vi "PatientSpecificFileNameGen.vi"(3 "Auto Increment":bool, 4 "Done":bool, 5 "Add to Database":bool) -> (0 "SavePathOut":path, 1 "PatientFileName":string)   [LabVIEW 2022 SP3]
uses:
  Patient Routines/PatientGlobals.vi
  ScanningControl/Motion Controllers/-MotionRoutines/MotionGlobals.vi
  ViewData/-ReadEye/TypeDefs/TissueType.ctl
  Patient Routines/LymphNodeInfo.ctl
  Patient Routines/TissueTypeScan.ctl
panel:
  in  "Node Info":T1 {"Year" format="%02d"; "Patient Number" format="%03d"; "Node Number" format="%02d"}
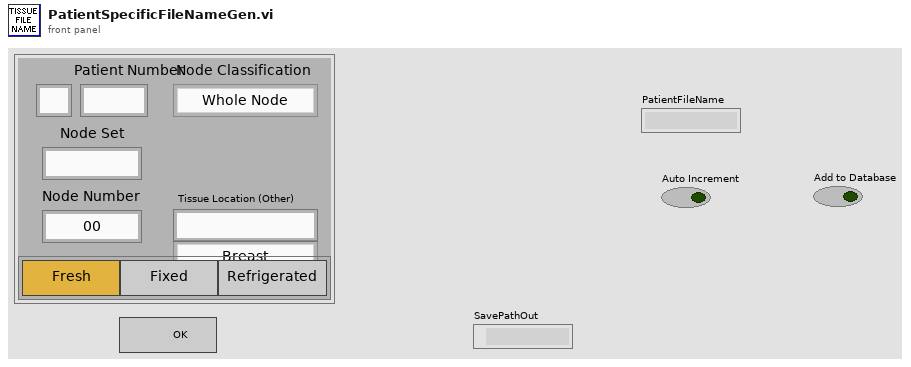
[diagram p1: front panel]
types:
  T1 = typedef "LymphNodeInfo.ctl" = cluster{"Patient Number":u32, "Node Set":string, "Node Number":u32, "Tissue Type":T2, "Tissue Location (Other)":string, "Node Classification":enum16{"Whole Node", "Piece A", "Piece B", "Piece C"}, "Fresh?":enum32{"Fresh?", "Fixed?", "Refrigerated?"}, "Year":u32}
  T2 = typedef "TissueTypeScan.ctl" = enum16{"Breast", "Gastric", "Stomach", "Rectal", "Colon", "Head & Neck", "Other"}
  T3 = typedef "location.ctl" = enum16{"Automatic", "WCM Main", "Hawaii", "Columbia MM3000", "Columbia  NI System", "NYU", "RRI 2", "UHI Allen", "CUMC RT", "Chiba", "Stony Brook", "WCM Microscopy", "WCM Aeoretch", "WCM Optics Lab", "WCM Main 2Axis", "WCM Rotation", "WCM SAM SMAC", "SERI GP"}
  T4 = enum16{"Whole Node", "Sentinel A", "Sentinel B", "Sentinel C"}
  T5 = typedef "TissueType.ctl" = enum16{"Breast", "Gastric", "Stomach", "Rectal", "Colon", "Head & Neck", "Other"}
  T6 = enum16{"open", "replace", "create", "open or create", "replace or create", "replace or create with confirmation"}
  T7 = typedef "TissueType.ctl" = cluster{"organ":i16, "disease type":i16, "disease location":i16, "IQ_pts":u16, "RcvBuffer":u8, "RcvFrame":u16, "IQBuff":u8, "IQFrame":u16, "IQPage":u8}
  T8 = enum16{"Whole Node", "Piece A", "Piece B", "Piece C"}
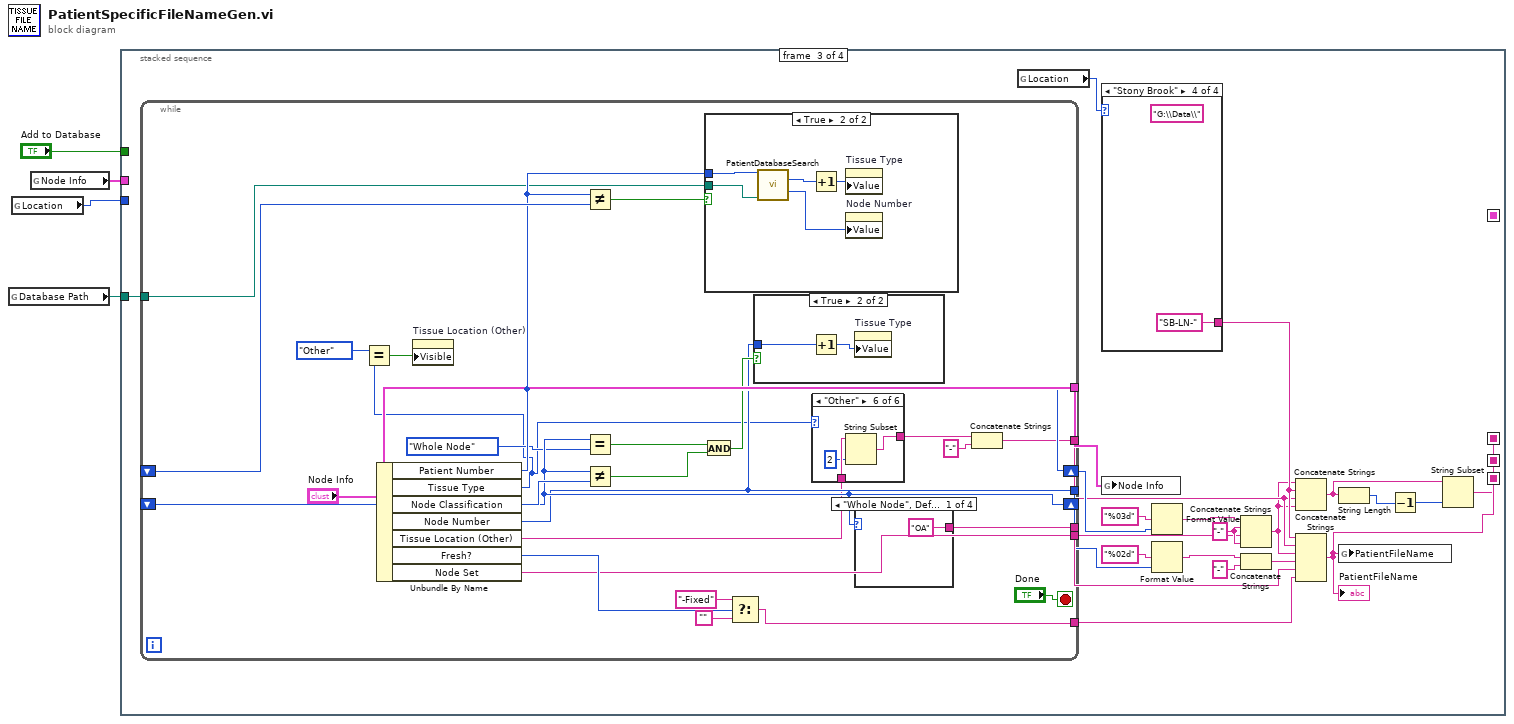
[diagram p0: block diagram]
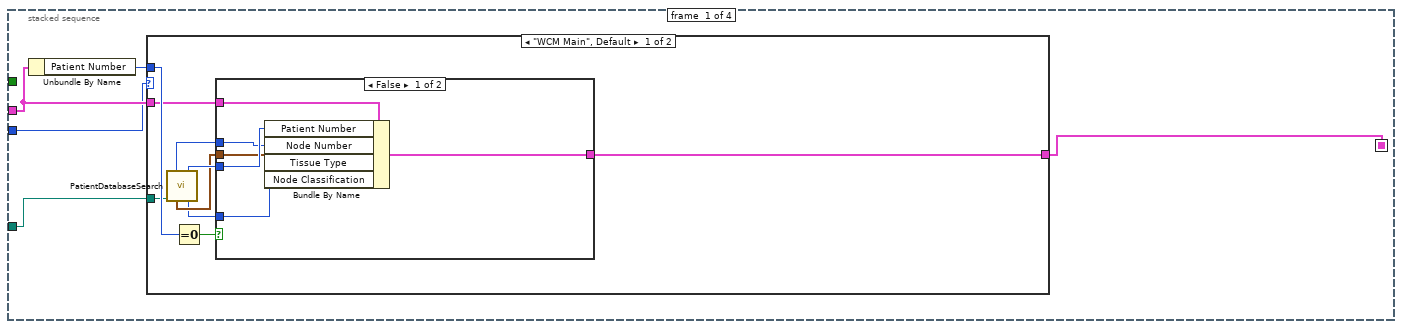
[diagram p2: hidden frame]
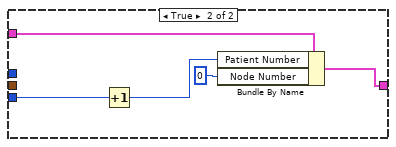
[diagram p3: hidden frame]
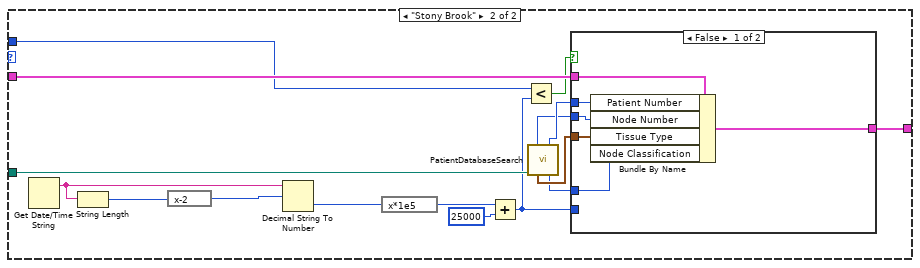
[diagram p4: hidden frame]
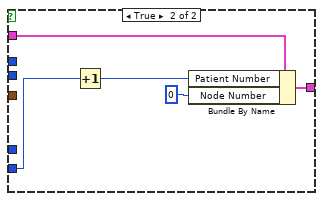
[diagram p5: hidden frame]
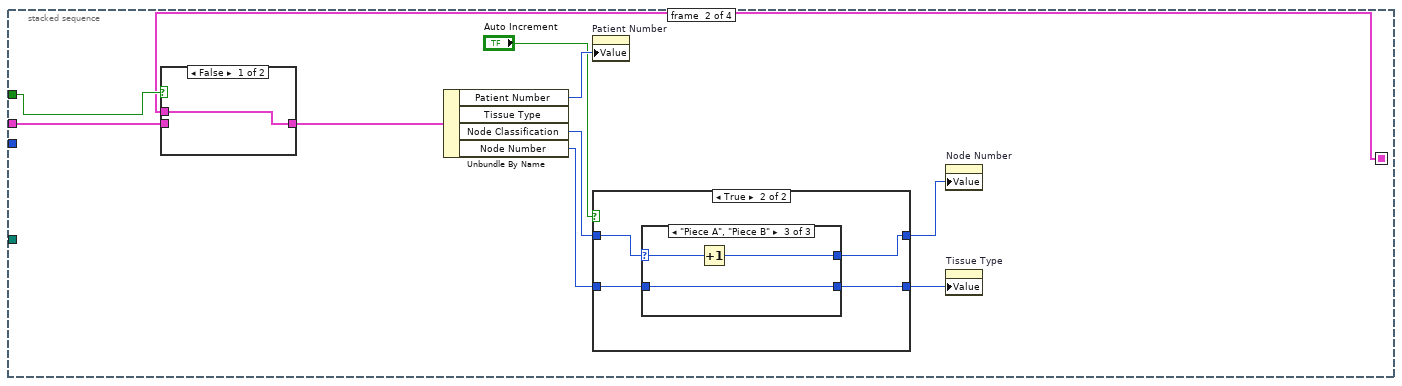
[diagram p6: hidden frame]
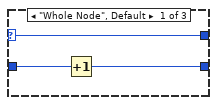
[diagram p9: hidden frame]
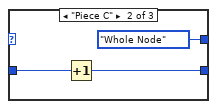
[diagram p10: hidden frame]
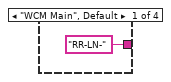
[diagram p11: hidden frame]
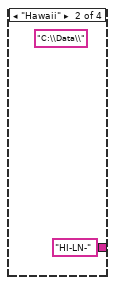
[diagram p12: hidden frame]
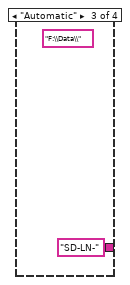
[diagram p13: hidden frame]
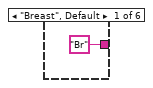
[diagram p16: hidden frame]
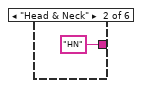
[diagram p17: hidden frame]
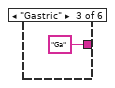
[diagram p18: hidden frame]
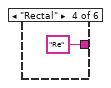
[diagram p19: hidden frame]
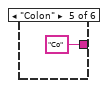
[diagram p20: hidden frame]
diagram:
  n1 = global read "PatientGlobals.vi" "Database Path"() -> (w4:path)
  n2 = global read "MotionGlobals.vi" "Location"() -> (w1:T3)
  n3 = global read "PatientGlobals.vi" "Node Info"() -> (w2:T1)
  n4 = stacked-sequence {
    seq-local: [_ _ w90 _] -> [_ _ _ w168]
    seq-local: [_ _ w101 _] -> [_ _ _ w166]
    seq-local: [_ _ w101 _] -> [_ _ _ w164]
    seq-local: [w6 _ _ _] -> [_ w57 _ _]
    tunnel: w4 -> [w8 _ w99 w163]
    tunnel: "Add to Database" -> [_ w60 _ w156]
    tunnel: w2 -> [w7 w59 _ _]
    tunnel: w1 -> [w5 _ _ _]
    frame #0 {
      n5 = Unbundle By Name(w7) -> ("Patient Number"=w9:u32)
      n6 = case shown="\"WCM Main\", Default" w5 {
        tunnel: w9 -> [w18 w38]
        tunnel: w8 -> [w16 w45]
        tunnel: w7 -> [w11 w40]
        tunnel: [w10 w39] -> w6
        frame "WCM Main", Default {
          n7 = call "PatientDatabaseSearch.vi"("file path (use dialog)"=w16) -> ("Last node of Last patient"=w14:i32, "Last Patient Number"=w15:i32, "Tissue Type of Last Node"=w13:T7, "Node Classification Of Last Patient"=w12:T4)  [unwired: 5 in, 6 out]
          n8 = Equal To 0?(x=w18) -> (x = 0?=w17:bool)
          n9 = case shown="False" w17 {
            tunnel: w11 -> [w24 w29]
            tunnel: w15 -> [w22 w27]
            tunnel: [w23 w25] -> w10
            tunnel: w14 -> [w21 _]
            tunnel: w13 -> [w20 _]
            tunnel: w12 -> [w19 _]
            frame False {
              n10 = Bundle By Name(cluster=w24, "Patient Number"=w22, "Node Number"=w21, "Tissue Type"=w20, "Node Classification"=w19) -> (w23:T1)
            }
            frame True {
              n11 = Increment(x=w27) -> (x+1=w28:i32)
              n12 = Bundle By Name(cluster=w29, "Patient Number"=w28, "Node Number"=u32 0) -> (w25:T1)
            }
          }
        }
        frame "Stony Brook" {
          n13 = Get Date/Time String() -> (date string=w35:string)  [unwired: 3 in, 1 out]
          n14 = String Length(string=w35) -> (length=w36:i32)
          n15 = expression code="x-2"(w36) -> (w34:i32)
          n16 = Decimal String To Number(string=w35, offset=w34) -> (number=w31:i32)  [unwired: 1 in, 1 out]
          n17 = expression code="x*1e5"(w31) -> (w30:i32)
          n18 = Add(x=w30, y=u32 25000) -> (x+y=w32:u32)
          n19 = Less?(x=w38, y=w32) -> (x < y?=w37:bool)
          n20 = call "PatientDatabaseSearch.vi"("file path (use dialog)"=w45) -> ("Last node of Last patient"=w43:i32, "Last Patient Number"=w44:i32, "Tissue Type of Last Node"=w42:T7, "Node Classification Of Last Patient"=w41:T4)  [unwired: 5 in, 6 out]
          n21 = case shown="False" w37 {
            tunnel: w40 -> [w51 w56]
            tunnel: w44 -> [w49 _]
            tunnel: [w50 w53] -> w39
            tunnel: w43 -> [w48 _]
            tunnel: w42 -> [w47 _]
            tunnel: w41 -> [w46 _]
            tunnel: w32 -> [_ w52]
            frame False {
              n22 = Bundle By Name(cluster=w51, "Patient Number"=w49, "Node Number"=w48, "Tissue Type"=w47, "Node Classification"=w46) -> (w50:T1)
            }
            frame True {
              n23 = Increment(x=w52) -> (x+1=w55:u32)
              n24 = Bundle By Name(cluster=w56, "Patient Number"=w55, "Node Number"=u32 0) -> (w53:T1)
            }
          }
        }
      }
    }
    frame #1 {
      n25 = case shown="False" w60 {
        tunnel: [w67 w68] -> w58
        tunnel: w59 -> [_ w68]
        tunnel: w57 -> [w67 _]
        frame False {
        }
        frame True {
        }
      }
      n26 = Unbundle By Name(w58) -> ("Patient Number"=w65:u32, "Node Classification"=w63:T8, "Node Number"=w64:u32)  [unwired: 1 out]
      n27 = property on="Patient Number" class="DigNum (strict)"("Value"=w65) -> ()  [unwired: 2 in, 2 out]
      n28 = case shown="True" "Auto Increment" {
        tunnel: [w69 w74] -> w66
        tunnel: w64 -> [w69 w73]
        tunnel: w63 -> [w70 w72]
        tunnel: [w70 w71] -> w62
        frame False {
        }
        frame True {
          n29 = case shown="\"Piece A\", \"Piece B\"" w72 {
            selector: w72 -> [w75 _ w82]
            tunnel: [w77 w78 w83] -> w74
            tunnel: w73 -> [w76 w79 w83]
            tunnel: [w75 T4."Whole Node" ("Node Classification") w81] -> w71
            frame "Whole Node", Default {
              n30 = Increment(x=w76) -> (x+1=w77:u32)
            }
            frame "Piece C" {
              n31 = Increment(x=w79) -> (x+1=w78:u32)
            }
            frame "Piece A", "Piece B" {
              n32 = Increment(x=w82) -> (x+1=w81:T8)
            }
          }
        }
      }
      n33 = property on="Node Number" class="DigNum (strict)"("Value"=w62) -> ()  [unwired: 2 in, 2 out]
      n34 = property on="Tissue Type" class="Enum (strict)"("Value"=w66) -> ()  [unwired: 2 in, 2 out]
    }
    frame #2 {
      w85 = "-" ("string")
      n35 = while {
        tunnel: [w121] -> w96
        tunnel: [w134] -> w102
        shift-right: [w130] -> w104
        shift-left: _ -> [w132]
        tunnel: ["Node Info"] -> w103
        tunnel: w99 -> [w129]
        shift-right: [w126] -> _
        shift-left: _ -> [w128]
        tunnel: [w122] -> w98
        tunnel: [w119] -> w86
        tunnel: [w116] -> w84
        stop <- "Done" stop-if-true
        n36 = Unbundle By Name("Node Info") -> ("Patient Number"=w130:u32, "Tissue Type"=w113:T2, "Node Classification"=w126:T8, "Node Number"=w122:u32, "Tissue Location (Other)"=w118:string, "Fresh?"=w120:enum32{"Fresh?", "Fixed?", "Refrigerated?"}, "Node Set"=w116:string)
        n37 = Equal?(x=TissueType."Other", y=w113) -> (x = y?=w112:bool)
        n38 = property on="Tissue Location (Other)" class="Str"("Visible"=w112) -> ()  [unwired: 2 in, 2 out]
        n39 = Not Equal?(x=w130, y=w132) -> (x != y?=w133:bool)
        n40 = Equal?(x=w126, y=T4."Whole Node" ("Node Classification")) -> (x = y?=w124:bool)
        n41 = Not Equal?(x=w126, y=w128) -> (x != y?=w127:bool)
        n42 = And(x=w124, y=w127) -> (x .and. y?=w123:bool)
        n43 = case shown="True" w133 {
          tunnel: w130 -> [_ w143]
          tunnel: w129 -> [_ w140]
          frame False {
          }
          frame True {
            n44 = call "PatientDatabaseSearch.vi"("Patient Info to Find"=w143, "file path (use dialog)"=w140) -> ("Last Node of Searched Patient"=w141:i32, "Node Classification Of Searched"=w139:T4)  [unwired: 4 in, 8 out]
            n45 = Increment(x=w141) -> (x+1=w142:i32)
            n46 = property on="Tissue Type" class="Enum (strict)"("Value"=w142) -> ()  [unwired: 2 in, 2 out]
            n47 = property on="Node Number" class="DigNum (strict)"("Value"=w139) -> ()  [unwired: 2 in, 2 out]
          }
        }
        n48 = Select(t="-Fixed" ("string"), s=w120, f="" ("t")) -> (s? t:f=w119:string)
        n49 = case shown="True" w123 {
          tunnel: w122 -> [_ w138]
          frame False {
          }
          frame True {
            n50 = Increment(x=w138) -> (x+1=w137:u32)
            n51 = property on="Tissue Type" class="Enum (strict)"("Value"=w137) -> ()  [unwired: 2 in, 2 out]
          }
        }
        n52 = case shown="\"Other\"" w113 {
          tunnel: ["Br" "HN" "Ga" "Re" "Co" w150] -> w135
          tunnel: w118 -> [_ _ _ _ _ w151]
          frame "Breast", Default {
          }
          frame "Head & Neck" {
          }
          frame "Gastric" {
          }
          frame "Rectal" {
          }
          frame "Colon" {
          }
          frame "Other" {
            n53 = String Subset(string=w151, length (rest)=2 ("length (rest)")) -> (substring=w150:string)  [unwired: 1 in]
          }
        }
        n54 = case shown="\"Whole Node\", Default" w126 {
          tunnel: ["OA" "SA" "SB" "SC"] -> w134
          frame "Whole Node", Default {
          }
          frame "Piece A" {
          }
          frame "Piece B" {
          }
          frame "Piece C" {
          }
        }
        n55 = Concatenate Strings(w135, "-" ("string")) -> (w121:string)
      }
      n56 = global read "MotionGlobals.vi" "Location"() -> (w100:T3)
      n57 = case shown="\"Stony Brook\"" w100 {
        tunnel: ["RR-LN-" "HI-LN-" "SD-LN-" "SB-LN-"] -> w97
        frame "WCM Main", Default {
        }
        frame "Hawaii" {
          (unwired) "C:\\Data\\"
        }
        frame "Automatic" {
          (unwired) "F:\\Data\\"
        }
        frame "Stony Brook" {
          (unwired) "G:\\Data\\"
        }
      }
      n58 = global write "PatientGlobals.vi" "Node Info"(w103) -> ()
      n59 = Format Value(format string="%03d", value (0)=w104) -> (output string=w95:string)  [unwired: 1 in]
      n60 = Format Value(format string="%02d", value (0)=w98) -> (output string=w92:string)  [unwired: 1 in]
      n61 = Concatenate Strings(w95, w85, w84, w85) -> (w94:string)
      n62 = Concatenate Strings(w92, "-" ("string")) -> (w91:string)
      n63 = Concatenate Strings(w94, w97, w96, w94) -> (w89:string)
      n64 = Concatenate Strings(w97, w96, w94, w91, w102, w86) -> (w101:string)
      "PatientFileName" <- w101
      n65 = String Length(string=w89) -> (length=w88:i32)
      n66 = global write "PatientGlobals.vi" "PatientFileName"(w101) -> ()
      n67 = Decrement(x=w88) -> (x-1=w87:i32)
      n68 = String Subset(string=w89, length (rest)=w87) -> (substring=w90:string)  [unwired: 1 in]
    }
    frame #3 {
      n69 = case shown="True" w156 {
        tunnel: w164 -> [_ w174]
        tunnel: w163 -> [_ w169]
        frame False {
        }
        frame True {
          n70 = call <vilib>:"Normalize End Of Line.vi"("string in"=w174) -> ("string out"=w180:string)  [unwired: 7 in]
          n71 = Concatenate Strings(w180, "\r") -> (w179:string)
          n72 = Open/Create/Replace File(file path (use dialog)=w169, operation (0:open)=T6."open or create") -> (refnum out=w175:refnum<file>, error out=w171:errorcluster)  [unwired: 4 in, 1 out]
          n73 = Read from Text File(file (use dialog)=w175, error in=w171) -> (refnum out=w173:refnum<file>, error out=w172:errorcluster)  [unwired: 2 in, 2 out]
          n74 = Write to Text File(file (use dialog)=w173, text=w179, error in=w172) -> (refnum out=w176:refnum<file>, error out=w177:errorcluster)  [unwired: 1 in, 1 out]
          n75 = Close File(refnum=w176, error in=w177) -> ()  [unwired: 2 out]
        }
      }
      n76 = global read "MotionGlobals.vi" "SavePath"() -> (w162:path)
      n77 = Path To String(path=w162) -> (string=w161:string)
      n78 = String Subset(string=w161, length (rest)=7 ("length (rest)")) -> (substring=w159:string)  [unwired: 1 in]
      n79 = String To Path(string=w159) -> (path=w158:path)
      n80 = Concatenate Strings(w168, "\\" ("string"), w166) -> (w165:string)
      n81 = Build Path(base path=w158, name or relative path=w165) -> (appended path=w157:path)
      "SavePathOut" <- w157
      n82 = global write "MotionGlobals.vi" "SavePath"(w157) -> ()
    }
  }
